vi "Renishaw-XL80_GetMeasurementMode.vi"(8 "error in (no error)":errorcluster, 11 "Renishaw-XL80_EMU in":refnum<class "Renishaw-XL80_EMU.lvclass">) -> (0 "error out":errorcluster, 2 "MeasurementMode":i32(ring) items=["MEASUREMENT_INDETERMINATE", "MEASUREMENT_LINEAR_PLANE", "MEASUREMENT_LINEAR_RETRO", "MEASUREMENT_ANGULAR", "MEASUREMENT_STRAIGHTNESS_SHORT", "MEASUREMENT_STRAIGHTNESS_LONG", "MEASUREMENT_VELOCITY_RETRO"], 3 "Renishaw-XL80_EMU out":refnum<class "Renishaw-XL80_EMU.lvclass">)   [LabVIEW 2024, in "Renishaw-XL80_EMU.lvclass"]
doc: "Reading this property retrieves the current measurement mode.\n\nDefinition\nHRESULTget_MeasurementMode( [out, retval] MEASUREMENT_MODES *pVal);\nParameters\npVal\nA variable that will be set to one of the value in the enumerated type MEASUREMENT_MODES\n\nComments\nReading this property will always retrieve the current measurement mode. This mode is the client's requested mode. It may not correspond to the measurement mode returned in the ML10 status, if for instance the ML10 has stopped responding.\n\nThe property will normally return an HRESULT of S_OK. However, it will return E_POINTER if the client supplies a null pointer for pVal.\nThis enumerated type defines constants that specify the measurement mode.\n\nDefinition\n[v1_enum]typedef enum MEASUREMENT_MODES { MEASUREMENT_INDETERMINATE = 0, MEASUREMENT_LINEAR_PLANE = 1, MEASUREMENT_LINEAR_RETRO = 2, MEASUREMENT_ANGULAR = 3, MEASUREMENT_STRAIGHTNESS_SHORT = 4, MEASUREMENT_STRAIGHTNESS_LONG = 5} MEASUREMENT_MODES;\nComments\nThe v1_enum attribute indicates that the enumerated type will be transmitted as a 32-bit entity.\n\nMEASUREMENT_INDETERMINATE may be returned as part of the ML10 status. This would indicate that the ML10 is not responding. Attempting to use this value to set the measurement mode will fail. \nMEASUREMENT_LINEAR_PLANE indicates that the reading is treated as linear using a plane mirror. \nMEASUREMENT_LINEAR_RETRO indicates that the reading is treated as linear using a retro-reflector. \nMEASUREMENT_ANGULAR indicates that the reading is treated as angular. \nMEASUREMENT_STRAIGHTNESS_SHORT indicates that the reading is treated as straightness using short range optics. \nMEASUREMENT_STRAIGHTNESS_LONG indicates that the reading is treated as straightness using long range optics."
uses:
  Renishaw-XL80_EMU.lvclass
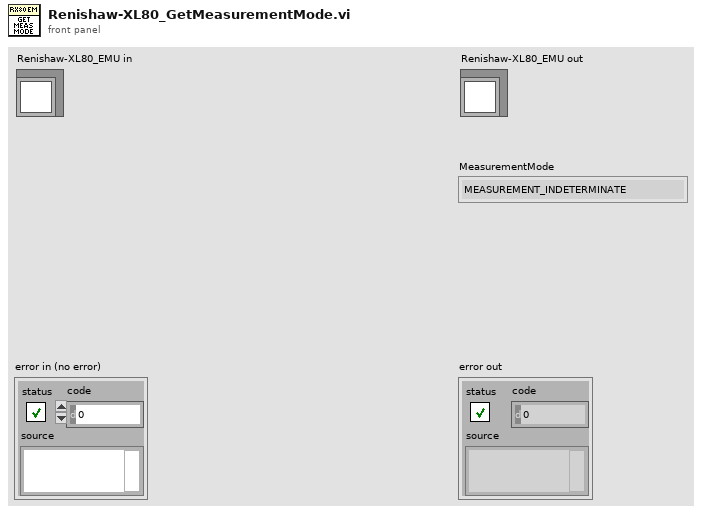
[diagram p1: front panel]
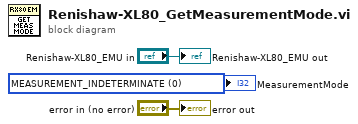
[diagram p0: block diagram]
diagram:
  w1 = 0 items=["MEASUREMENT_INDETERMINATE", "MEASUREMENT_LINEAR_PLANE", "MEASUREMENT_LINEAR_RETRO", "MEASUREMENT_ANGULAR", "MEASUREMENT_STRAIGHTNESS_SHORT", "MEASUREMENT_STRAIGHTNESS_LONG", "MEASUREMENT_VELOCITY_RETRO"] ("MeasurementMode")
  "error out" <- "error in (no error)"
  "Renishaw-XL80_EMU out" <- "Renishaw-XL80_EMU in"
  "MeasurementMode" <- w1
